vi "writeToXML.vi"(8 "error in (no error)":errorcluster, 10 "ClassLabel":string, 11 "TCSWFSCommand in":refnum<class "TCSWFSCommand.lvclass">) -> (0 "error out":errorcluster, 2 "XMLout":string, 3 "TCSWFSCommand out":refnum<class "TCSWFSCommand.lvclass">)   [LabVIEW 2014, in "TCSDataDefinitions.lvlib" / "TCSWFSCommand.lvlib" / "TCSWFSCommand.lvclass"]
uses:
  TCSWFSCommand.lvclass
  TCSCommand/TCSCommand/TCSCommand.lvclass
  <userlib>/Common/XML/XMLGenerator/XMLGenerator.lvclass
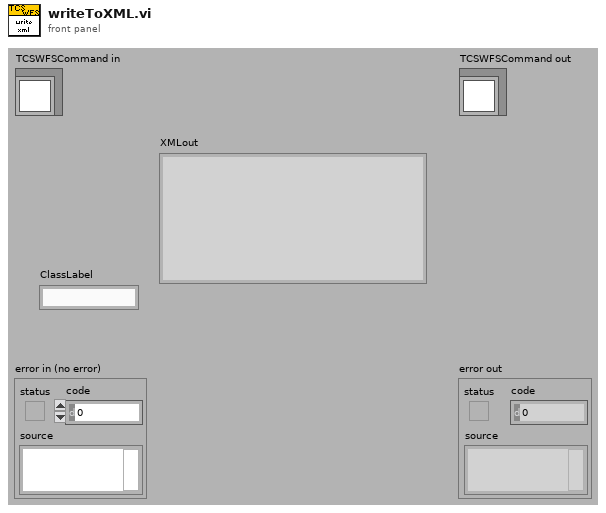
[diagram p1: front panel]
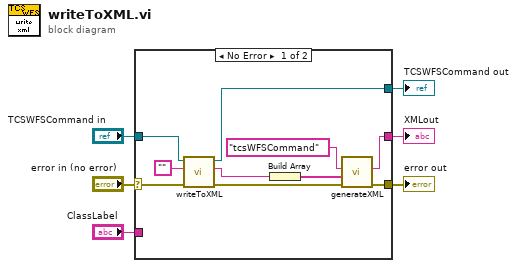
[diagram p0: block diagram]
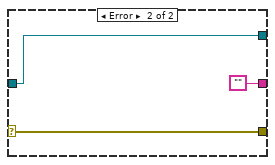
[diagram p2: hidden frame]
diagram:
  n1 = case shown="No Error" "error in (no error)" {
    selector: "error in (no error)" -> [w15 w19]
    tunnel: [w10 w19] -> w5
    tunnel: [w7 w18] -> w3
    tunnel: "TCSWFSCommand in" -> [w8 w18]
    tunnel: [w9 ""] -> w2
    tunnel: "ClassLabel" -> [_ _]
    frame No Error {
      n2 = call-parent "writeToXML.vi"("error in (no error)"=w15, "Class Label"="", "TCSCommand in"=w8) -> ("error out"=w11:errorcluster, "XML out"=w14:string, "TCSCommand out"=w7:refnum<class "TCSWFSCommand.lvclass">)  [unwired: 6 in]
      n3 = Build Array(w14) -> (w13:string[])
      n4 = call <userlib>:"generateXML.vi"("error in"=w11, "childrenXML"=w13, "elementName"="tcsWFSCommand" ("Class Label")) -> ("error out"=w10:errorcluster, "XML out"=w9:string)  [unwired: 6 in, 1 out]
    }
    frame Error {
    }
  }
  "error out" <- w5
  "TCSWFSCommand out" <- w3
  "XMLout" <- w2
